vi "ControlShutter.vi"() -> ()   [LabVIEW 2023]
panel:
  out "error out 2":errorcluster
  in  "Voltage 2":u16
  in  "stop 2":bool
  out "error out":errorcluster
  in  "stop":bool
  in  "Voltage":u16
  in  "VISA Refnum in":refnum<visa-resource-name>
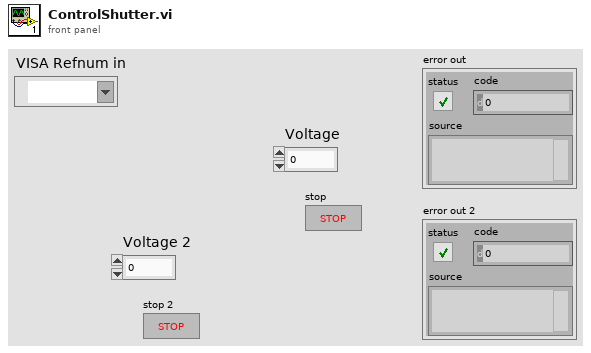
[diagram p1: front panel]
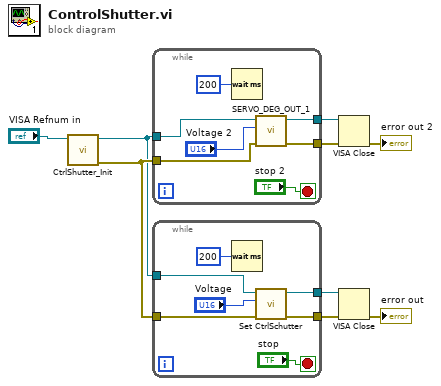
[diagram p0: block diagram]
diagram:
  n1 = call "CtrlShutter_Init.vi"("VISA Refnum in"="VISA Refnum in") -> ("error out"=w2:errorcluster, "VISA Refnum out"=w1:refnum<visa-resource-name>)  [unwired: 8 in, 1 out]
  n2 = while {
    tunnel: w1 -> [w14]
    tunnel: w2 -> [w12]
    tunnel: [w10] -> w6
    tunnel: [w11] -> w5
    stop <- "stop 2" stop-if-true
    n3 = Wait (ms)(milliseconds to wait=u32 200) -> ()  [unwired: 1 out]
    n4 = call "SERVO_DEG_OUT_1.vi"("VISA Refnum in"=w14, "Voltage"="Voltage 2", "error in (no error)"=w12) -> ("VISA Refnum out"=w10:refnum<visa-resource-name>, "error out"=w11:errorcluster)  [unwired: 5 in, 1 out]
  }
  n5 = while {
    tunnel: w1 -> [w23]
    tunnel: w2 -> [w22]
    tunnel: [w18] -> w9
    tunnel: [w17] -> w8
    stop <- "stop" stop-if-true
    n6 = Wait (ms)(milliseconds to wait=u32 200) -> ()  [unwired: 1 out]
    n7 = call "Set CtrlSchutter.vi"("VISA Refnum in"=w23, "Voltage"="Voltage", "error in (no error)"=w22) -> ("VISA Refnum out"=w18:refnum<visa-resource-name>, "error out"=w17:errorcluster)  [unwired: 5 in, 1 out]
  }
  n8 = VISA Close(VISA resource name=w6, error in (no error)=w5) -> (error out=→"error out 2":errorcluster)
  n9 = VISA Close(VISA resource name=w9, error in (no error)=w8) -> (error out=→"error out":errorcluster)
